vi "Global  HARDWARE.vi"() -> ()   [LabVIEW 2019]
uses:
  Controls/def MOTOR info.ctl
  Controls/ctrl MOTOR CTRLR SELECT.ctl
  <vilib>/Rock Robotics/SystemInterfaces/DIO/FPGA_DIOPWMChannel.ctl
  <vilib>/Rock Robotics/WPI/ThirdParty/REV Robotics/SPARK MAX/Typedef/Spark MAX Motor Type.ctl
  Controls/def ENCODER info.ctl
  <vilib>/Rock Robotics/SystemInterfaces/DIO/FPGA_DIOChannel.ctl
  <vilib>/Rock Robotics/WPI/Encoder/WPI_EncoderType.ctl
  Controls/def GYRO info.ctl
  <vilib>/Rock Robotics/SystemInterfaces/spilib/spi_bus.ctl
  Controls/ctrl ANALOG CHANNEL SELECT.ctl
  Controls/def SONAR info.ctl
  Controls/ctrl SONAR DEVICE SELECT.ctl
  <vilib>/Rock Robotics/WPI/Ultrasonic/WPI_UltrasonicRangeUnits.ctl
  Controls/def SERVO info.ctl
  Controls/def USER CONTROL info.ctl
  <vilib>/Rock Robotics/WPI/Joystick/WPI_JoystickDeviceEnum.ctl
  Controls/def JOYSTICK PARAMETERS.ctl
  Controls/ctrl ENCODER SELECT.ctl
  Controls/ctrl MOTOR SELECT.ctl
  Controls/ctrl SERVO SELECT.ctl
  Controls/ctrl SONAR SELECT.ctl
  Controls/ctrl JOYSTICK CTRLR SELECT.ctl
  Controls/def COMPRESSOR info.ctl
  Controls/def AIR PRESSURE info.ctl
  <vilib>/Rock Robotics/SystemInterfaces/AI/FPGA_AIChannel.ctl
  Controls/ctrl AIRPRESS SELECT.ctl
  Controls/def SOLENOID info.ctl
  <vilib>/Rock Robotics/WPI/Solenoid/WPI_SolenoidChannel.ctl
  <vilib>/Rock Robotics/WPI/Solenoid/WPI_SolenoidValue.ctl
  Controls/def RELAY info.ctl
  <vilib>/Rock Robotics/SystemInterfaces/DIO/FPGA_DIORelayChannel.ctl
  <vilib>/Rock Robotics/WPI/Relay/WPI_RelayDirection.ctl
  <vilib>/Rock Robotics/WPI/Relay/WPI_RelayValue.ctl
  Controls/def LIMIT SWITCH info.ctl
  Controls/ctrl LOOP TIMES def.ctl
  Controls/ctrl SOLENOID SELECT.ctl
panel:
  in  "Tab Control":T1(tab)=enum."DRIVE TRAIN"
  in  "AUTO selector names":string[](array[string])=["PGM ARRAY", "--", "--", "TEST DRIVE MOTOR REACTIONS"]
  in  "String names":string[](array[string])=["Column hdr 1", "---", "----", "----", "----", "Column hdr 2", "---", "---", "---", "---"]
  in  "LED names":string[](array[string])=["LED 0", "LED 1", "LED 2", "LED 3"]
  in  "Slider names":string[](array[string])=["SLDR 0", "SLDR 1", "SLDR 2", "SLDR 3"]
  in  "Button names":string[](array[string])=["BTN 0", "BTN 1", "BTN 2", "BTN 3"]
  in  "START-UP String":cluster{"stack name":string, "String":string}[](array[cluster])=[{"stack name"="", "String"=""}]
  in  "START-UP Boolean":cluster{"stack name":string, "value":bool}[](array[cluster])=[{"stack name"="shooter switch", "value"=TRUE}]
  in  "START-UP Number":cluster{"stack name":string, "value":dbl}[](array[cluster])=[{"stack name"="Shooter Speed", "value"=0.7}, {"stack name"="Scoop Speed", "value"=0.7}, {"stack name"="agitator", "value"=1.0}]
  in  "LOOPING TIMERS":T2={"Input controllers"=25, "Drive system"=25, "Encoders"=25, "Limit switches"=25, "Sonar"=25, "Servos"=25, "Gyro"=25, "AIR PRESS"=25, "Solenoids"=25, "Motors"=25} {"Motors" min=10 step=5; "Solenoids" min=10 step=5; "AIR PRESS" min=10 step=5; "Gyro" min=10 step=5; "Servos" min=10 step=5; "Sonar" min=10 step=5; "Limit switches" min=10 step=5; "Encoders" min=10 step=5; "Drive system" min=10 step=5; "Input controllers" min=10 step=5}
  in  "SELECT INPUT CONTROL":T3 items=["Joystick 0"]
  in  "Controller":T4[](array[typedef])=[{"Descr"="Joystick", "Installed?"=TRUE, "RefName"="Joystick 0", "JoystickDevice"=enum."USB 0", "Invert Y axis"=FALSE, "Scale"=127.0, "AXIS"="Joysick 0/Axes", "BUTTONS"="Joysick 0/Buttons", "POV"="Joysick 0/POV", "Parameters"={"MAX LIMIT"=0.8, "MIN SPEED"=0.25, "DEADBAND"=0.05, "invert X?"=FALSE, "invert Y?"=FALSE}}] {"Parameters"."DEADBAND" format="%#_13g"; "Parameters"."MIN SPEED" format="%#_13g"; "Parameters"."MAX LIMIT" format="%#_13g"}
  in  "DRIVE CONFIGURATION":string(combo)="2 DRIVES x 2 MOTORS"
  in  "DRIVE MOTORS":T7[](array[typedef])=[{"Descr"="DRIVE LEFT1", "Motor Controller"=8, "PWM ch"=enum."Invalid", "Invert?"=FALSE, "Installed?"=TRUE, "RefName"="DRIVE_LEFT1", "stack name"="DRIVE/LEFT1", "remove deadband"=FALSE, "CAN ID"=1, "IDLE BEHAVIOUR"="COAST", "Motor Type"=enum."Brushless"}, {"Descr"="DRIVE LEFT2", "Motor Controller"=8, "PWM ch"=enum."Invalid", "Invert?"=FALSE, "Installed?"=TRUE, "RefName"="DRIVE_LEFT2", "stack name"="DRIVE/LEFT2", "remove deadband"=FALSE, "CAN ID"=2, "IDLE BEHAVIOUR"="COAST", "Motor Type"=enum."Brushless"}, {"Descr"="DRIVE_RIGHT1", "Motor Controller"=8, "PWM ch"=enum."Invalid", "Invert?"=TRUE, "Installed?"=TRUE, "RefName"="DRIVE_RT1", "stack name"="DRIVE/RIGHT1", "remove deadband"=FALSE, "CAN ID"=3, "IDLE BEHAVIOUR"="COAST", "Motor Type"=enum."Brushless"}, {"Descr"="DRIVE_RIGHT2", "Motor Controller"=8, "PWM ch"=enum."Invalid", "Invert?"=TRUE, "Installed?"=TRUE, "RefName"="DRIVE_RT2", "stack name"="DRIVE/RIGHT2", "remove deadband"=FALSE, "CAN ID"=4, "IDLE BEHAVIOUR"="COAST", "Motor Type"=enum."Brushless"}] {"CAN ID" min=1 max=62 step=1; "Motor Controller" items=["SPARK", "Existing", "SD540", "TALON SRX", "VICTOR SP", "TALON SR", "JAGUAR", "VICTOR", "SPARK MAX"]}
  in  "SELECT MOTOR":T11 items=["none"]
  in  "MOTORS":T7[](array[typedef]) {"CAN ID" min=1 max=62 step=1; "Motor Controller" items=["SPARK", "Existing", "SD540", "TALON SRX", "VICTOR SP", "TALON SR", "JAGUAR", "VICTOR"]}
  in  "SELECT SERVO":T12 items=["CAMERA", "SHOOTER", "BALL AGITATOR"]
  in  "SERVOS":T13[](array[typedef])
  in  "GYRO HARDWARE":T14={"Descr"="GYRO", "Installed?"=FALSE, "SPI Bus"=enum."Invalid", "AnalogChannel"=enum."AI 1", "Calibrate On Open"=TRUE, "Calibrated Center Voltage"=0.0, "Calibration Time (s)"=2.0, "Sample Rate (Hz)"=100.0, "RefName"="GYRO", "stack name"="GYRO"}
  in  "SELECT SOLENOID":T17 items=["none"]
  in  "SOLENOID":T18[](array[typedef])
  in  "SELECT AIR SENSOR":T21 items=["none"]
  in  "AIR PRESSURE":T22[](array[typedef]) {"warning HIGH" format="%.2f"; "warning LOW" format="%.2f"; "nominal value" format="%.2f"}
  in  "COMPRESSOR":T24={"Descr"="COMPRESSOR", "Installed?"=FALSE, "Pneumatics Control Module"=0, "RefName"="COMPRESSOR", "stack name"="COMPRESSOR"}
  in  "SELECT ENCODER":T25 items=["LEFT DRIVE MOTOR", "RIGHT DRIVE MOTOR", "MAST ENCODER"]
  in  "ENCODERS":T26[](array[typedef])=[{"Descr"="ENCODER DRIVE LEFT", "Installed?"=TRUE, "A Channel"=enum."DIO 5", "B Channel"=enum."DIO 6", "Invert Direction"=TRUE, "Enum"=enum."4x", "Gear ratio"=1.0, "Cycles per Rev"=1024.0, "Diameter (in)"=0.1016, "RefName"="ENC_L", "stack name"="DB/DRIVE/ENC-L", "min rate (hz)"=2.0, "Samples"=2, "STACK subnames"={"RESET name"="/reset", "STOPPED name"="/stopped", "DIRECTION name"="/direction", "RATE name"="/rate", "INSTALLED name"="/installed"}}, {"Descr"="ENCODER DRIVE RIGHT", "Installed?"=TRUE, "A Channel"=enum."DIO 3", "B Channel"=enum."DIO 4", "Invert Direction"=FALSE, "Enum"=enum."4x", "Gear ratio"=1.0, "Cycles per Rev"=1024.0, "Diameter (in)"=0.1016, "RefName"="ENC_R", "stack name"="DB/DRIVE/ENC-R", "min rate (hz)"=2.0, "Samples"=2, "STACK subnames"={"RESET name"="/reset", "STOPPED name"="/stopped", "DIRECTION name"="/direction", "RATE name"="/rate", "INSTALLED name"="/installed"}}]
  in  "RELAY":T29[](array[typedef])
  in  "LIMIT":T33[](array[typedef])
  in  "SELECT SONAR SOURCE":T34 items=["none"]
  in  "SONAR":T35[](array[typedef])
  in  "TESTMODE PROGRESS 0-100":string="TestMode/TestProgress"
  in  "TESTMODE PROGESS TEXT":string="TestMode/TestProgressText"
  in  "TESTMODE NAME":string="TestMode/TestName"
  in  "Default Tests":string[](array[string])=["Example Test", "test drive reactions", "List of tests is built in robot code.", "Replace with your own automated tests."]
  # "write this list to \"Auto List\" network stack... NOT \"DB/Auto List\"\nDASHBOARD will automatically be populated but Autonomous\nwill not; you will need to modify the Autonomous select cases\nmanually. They must match precisely.\nDASHBOARD will write \"Auto Selector\" with the selected auto\npgm chosen."
  # "only index 0 and 5 are seen as\nlabels over string columns"
  # "IMPORTANT:\nIn a 2-drive system, make LEFT index 0; RIGHT index 1.\nIn a 4-drive system, make REAR LEFT index 0; REAR RIGHT index 1; FRONT LEFT index 2; FRONT RIGHT index 3"
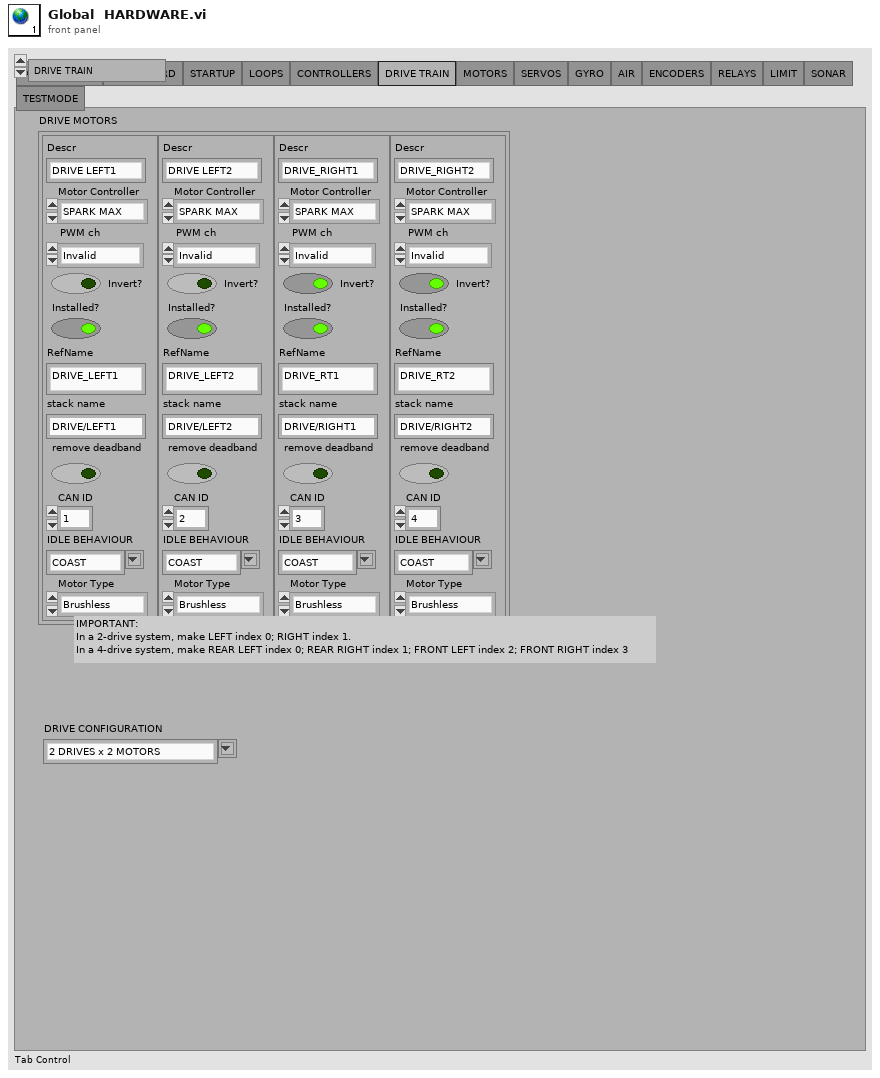
[diagram p1: front panel]
types:
  T1 = enum32{"AUTONOMOUS", "DASHBOARD", "STARTUP", "LOOPS", "CONTROLLERS", "DRIVE TRAIN", "MOTORS", "SERVOS", "GYRO", "AIR", "ENCODERS", "RELAYS", "LIMIT", "SONAR", "TESTMODE"}
  T2 = typedef "ctrl LOOP TIMES def.ctl" = cluster{"Input controllers":u8, "Drive system":u8, "Encoders":u8, "Limit switches":u8, "Sonar":u8, "Servos":u8, "Gyro":u8, "AIR PRESS":u8, "Solenoids":u8, "Motors":u8}
  T3 = typedef "ctrl JOYSTICK CTRLR SELECT.ctl" = u16
  T4 = typedef "def USER CONTROL info.ctl" = cluster{"Descr":string, "Installed?":bool, "RefName":string, "JoystickDevice":T5, "Invert Y axis":bool, "Scale":dbl, "AXIS":string, "BUTTONS":string, "POV":string, "Parameters":T6}
  T5 = typedef "WPI_JoystickDeviceEnum.ctl" = enum16{"USB 0", "USB 1", "USB 2", "USB 3", "USB 4", "USB 5"}
  T6 = typedef "def JOYSTICK PARAMETERS.ctl" = cluster{"MAX LIMIT":dbl, "MIN SPEED":dbl, "DEADBAND":dbl, "invert X?":bool, "invert Y?":bool}
  T7 = typedef "def MOTOR info.ctl" = cluster{"Descr":string, "Motor Controller":T8, "PWM ch":T9, "Invert?":bool, "Installed?":bool, "RefName":string, "stack name":string, "remove deadband":bool, "CAN ID":u8, "IDLE BEHAVIOUR":string, "Motor Type":T10}
  T8 = typedef "ctrl MOTOR CTRLR SELECT.ctl" = u16
  T9 = typedef "FPGA_DIOPWMChannel.ctl" = enum8{"PWM 0", "PWM 1", "PWM 2", "PWM 3", "PWM 4", "PWM 5", "PWM 6", "PWM 7", "PWM 8", "PWM 9", "PWM MXP 0", "PWM MXP 1", "PWM MXP 2", "PWM MXP 3", "PWM MXP 4", "PWM MXP 5", "PWM MXP 6", "PWM MXP 7", "PWM MXP 8", "PWM MXP 9", "Invalid"}
  T10 = typedef "Spark MAX Motor Type.ctl" = enum16{"Brushed", "Brushless"}
  T11 = typedef "ctrl MOTOR SELECT.ctl" = u16
  T12 = typedef "ctrl SERVO SELECT.ctl" = u16
  T13 = typedef "def SERVO info.ctl" = cluster{"Descr":string, "PWM ch":T9, "Installed?":bool, "Angular range":dbl, "RefName":string, "stack name":string}
  T14 = typedef "def GYRO info.ctl" = cluster{"Descr":string, "Installed?":bool, "SPI Bus":T15, "AnalogChannel":T16, "Calibrate On Open":bool, "Calibrated Center Voltage":dbl, "Calibration Time (s)":dbl, "Sample Rate (Hz)":dbl, "RefName":string, "stack name":string}
  T15 = typedef "spi_bus.ctl" = enum16{"SPI On-Board, CS0", "SPI On-Board, CS1", "SPI On-Board, CS2", "SPI On-Board, CS3", "SPI MXP", "Invalid"}
  T16 = typedef "ctrl ANALOG CHANNEL SELECT.ctl" = enum8{"AI 0", "AI 1", "Invalid"}
  T17 = typedef "ctrl SOLENOID SELECT.ctl" = u16
  T18 = typedef "def SOLENOID info.ctl" = cluster{"Descr":string, "Installed?":bool, "Pneumatics Control Module (0)":u8, "DBL":bool, "SolenoidChannel":T19, "SolenoidChannel":T19, "Default SET":T20, "RefName":string, "Value":string}
  T19 = typedef "WPI_SolenoidChannel.ctl" = enum8{"Solenoid 0", "Solenoid 1", "Solenoid 2", "Solenoid 3", "Solenoid 4", "Solenoid 5", "Solenoid 6", "Solenoid 7", "Invalid"}
  T20 = typedef "WPI_SolenoidValue.ctl" = enum16{"Off", "On", "Forward", "Reverse"}
  T21 = typedef "ctrl AIRPRESS SELECT.ctl" = u16
  T22 = typedef "def AIR PRESSURE info.ctl" = cluster{"Descr":string, "Installed?":bool, "Channel":T23, "RefName":string, "stack name":string, "MULTIPLIER":dbl, "OFFSET":dbl, "nominal value":dbl, "warning LOW":dbl, "warning HIGH":dbl}
  T23 = typedef "FPGA_AIChannel.ctl" = enum8{"AI 0", "AI 1", "AI 2", "AI 3", "AI MXP 0", "AI MXP 1", "AI MXP 2", "AI MXP 3", "Invalid"}
  T24 = typedef "def COMPRESSOR info.ctl" = cluster{"Descr":string, "Installed?":bool, "Pneumatics Control Module":u8, "RefName":string, "stack name":string}
  T25 = typedef "ctrl ENCODER SELECT.ctl" = u16
  T26 = typedef "def ENCODER info.ctl" = cluster{"Descr":string, "Installed?":bool, "A Channel":T27, "B Channel":T27, "Invert Direction":bool, "Enum":T28, "Gear ratio":dbl, "Cycles per Rev":dbl, "Diameter (in)":dbl[unit], "RefName":string, "stack name":string, "min rate (hz)":dbl, "Samples":u8, "STACK subnames":cluster{"RESET name":string, "STOPPED name":string, "DIRECTION name":string, "RATE name":string, "INSTALLED name":string}}
  T27 = typedef "FPGA_DIOChannel.ctl" = enum8{"DIO 0", "DIO 1", "DIO 2", "DIO 3", "DIO 4", "DIO 5", "DIO 6", "DIO 7", "DIO 8", "DIO 9", "DIO MXP 0", "DIO MXP 1", "DIO MXP 2", "DIO MXP 3", "DIO MXP 4", "DIO MXP 5", "DIO MXP 6", "DIO MXP 7", "DIO MXP 8", "DIO MXP 9", "DIO MXP 10", "DIO MXP 11", "DIO MXP 12", "DIO MXP 13", "DIO MXP 14", "DIO MXP 15", "SPI Port CS1", "SPI Port CS2", "SPI Port CS3", "SPI Port MISO", "SPI Port MOSI", "Invalid"}
  T28 = typedef "WPI_EncoderType.ctl" = enum16{"1x", "2x", "4x"}
  T29 = typedef "def RELAY info.ctl" = cluster{"Descr":string, "Installed?":bool, "RelayChannel":T30, "Relay Direction":T31, "Relay Value":T32, "RefName":string, "Value":string}
  T30 = typedef "FPGA_DIORelayChannel.ctl" = enum8{"Relay 0", "Relay 1", "Relay 2", "Relay 3", "Invalid"}
  T31 = typedef "WPI_RelayDirection.ctl" = enum16{"Both directions", "Forward only", "Reverse only"}
  T32 = typedef "WPI_RelayValue.ctl" = enum16{"Off", "On", "Forward", "Reverse"}
  T33 = typedef "def LIMIT SWITCH info.ctl" = cluster{"Descr":string, "Installed?":bool, "A Channel":T27, "Normally Closed?":bool, "RefName":string, "stack name":string}
  T34 = typedef "ctrl SONAR SELECT.ctl" = u16
  T35 = typedef "def SONAR info.ctl" = cluster{"Descr":string, "Installed?":bool, "Device type":T36, "PING Channel":T27, "ECHO Channel":T27, "RefName":string, "stack name":string, "Samples":i32, "Range Units":T37}
  T36 = typedef "ctrl SONAR DEVICE SELECT.ctl" = enum16{"SRF04 Digital", "MB1010 Digital", "MB1010 Analog", "SRF08 Digital"}
  T37 = typedef "WPI_UltrasonicRangeUnits.ctl" = enum16{"inches", "mm"}
diagram:
